vi "Ejercicio_07_Histograma.vi"() -> ()   [LabVIEW 2020]
uses:
  <vilib>/Instr/_visa.llb/VISA Configure Serial Port (Instr).vi
  <vilib>/Analysis/NI_AALBase.lvlib
panel:
  in  "VISA resource name 2":refnum<visa-resource-name>
  out "read buffer":string
  in  "stop":bool
  out "Histogram Graph":T1(graph)
  out "number":i64
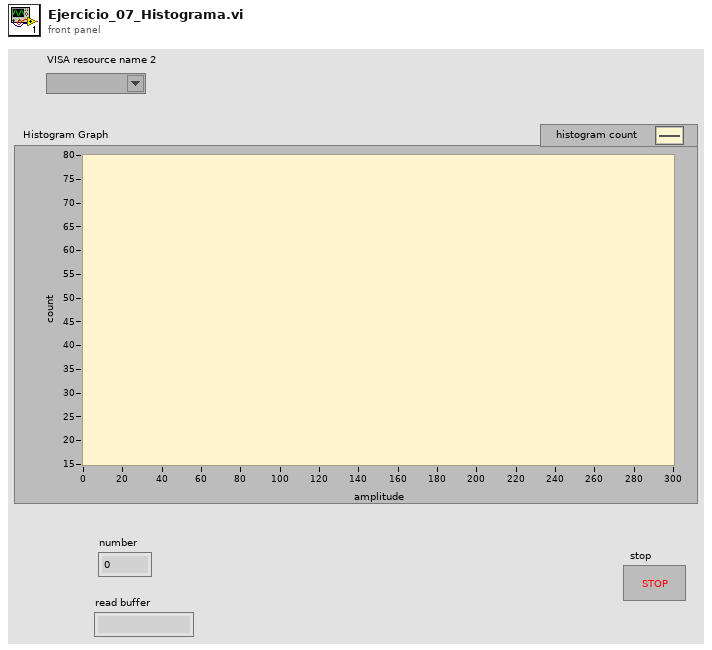
[diagram p1: front panel]
types:
  T1 = cluster{"X Values":dbl[], "Histogram: h(x)":i32[]}
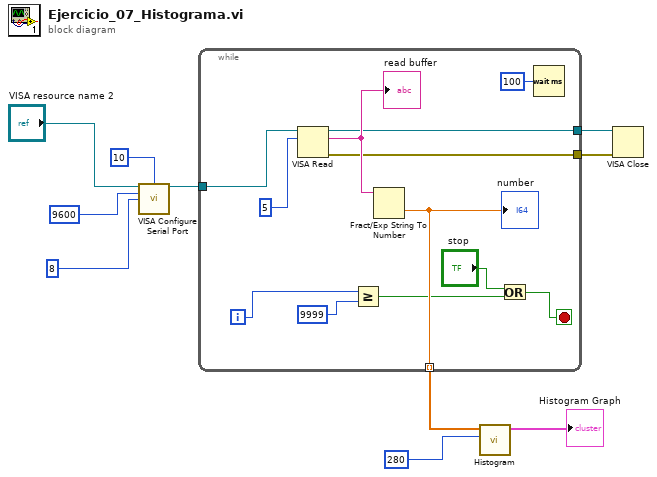
[diagram p0: block diagram]
diagram:
  n1 = call-poly "VISA Configure Serial Port"("VISA resource name"="VISA resource name 2", "termination char\n(0xA = '\\n' = LF)"=u32 10 ("timeout (10sec)"), "baud rate (9600)"=u32 9600 ("source offset (0)"), "data bits (8)"=u32 8 ("dest offset (0)")) -> ("VISA resource name out"=w7:refnum<visa-resource-name>)  [unwired: 10 in, 1 out]
  n2 = while {
    tunnel: [w21] -> w5 mode=indexing
    tunnel: w7 -> [w16]
    tunnel: [w13] -> w4
    tunnel: [w12] -> w3
    i -> [w20]
    stop <- w18 stop-if-true
    n3 = VISA Read(VISA resource name=w16, byte count=u32 5) -> (VISA resource name out=w13:refnum<visa-resource-name>, read buffer=w14:string, error out=w12:errorcluster)  [unwired: 1 in, 1 out]
    "read buffer" <- w14
    n4 = Greater Or Equal?(x=w20, y=9999) -> (x >= y?=w19:bool)
    n5 = Fract/Exp String To Number(string=w14) -> (number=w21:dbl)  [unwired: 3 in, 1 out]
    "number" <- w21
    n6 = Or(x="stop", y=w19) -> (x .or. y?=w18:bool)
    n7 = Wait (ms)(milliseconds to wait=u32 100) -> ()  [unwired: 1 out]
  }
  n8 = call <vilib>:"Histogram.vi"("intervals"=280, "X"=w5) -> ("Histogram Graph"=→"Histogram Graph":T1)  [unwired: 6 in, 3 out]
  n9 = VISA Close(VISA resource name=w4, error in (no error)=w3) -> ()  [unwired: 1 out]
